vi "main.vi"() -> ()   [LabVIEW 2013]
panel:
  out "Array 2":string[](array[string])
  in  "Tab Control":enum32{"Page 1", "Page 2"}(tab)
  in  "Ring 2":u16(ring)
  in  "Ring":u16(ring)
  out "XY Graph":cluster{"X":dbl, "Y":dbl}[](graph)
  out "Waveform Chart":dbl(graph)
  in  "Listbox":i32(listbox)
  in  "Cluster":cluster{"String":string}
  in  "Array":dbl[](array[numeric])
  out "String 2":string
  in  "String":string
  out "Boolean 2":bool
  out "Numeric 2":dbl
  in  "Boolean":bool
  in  "Numeric":dbl
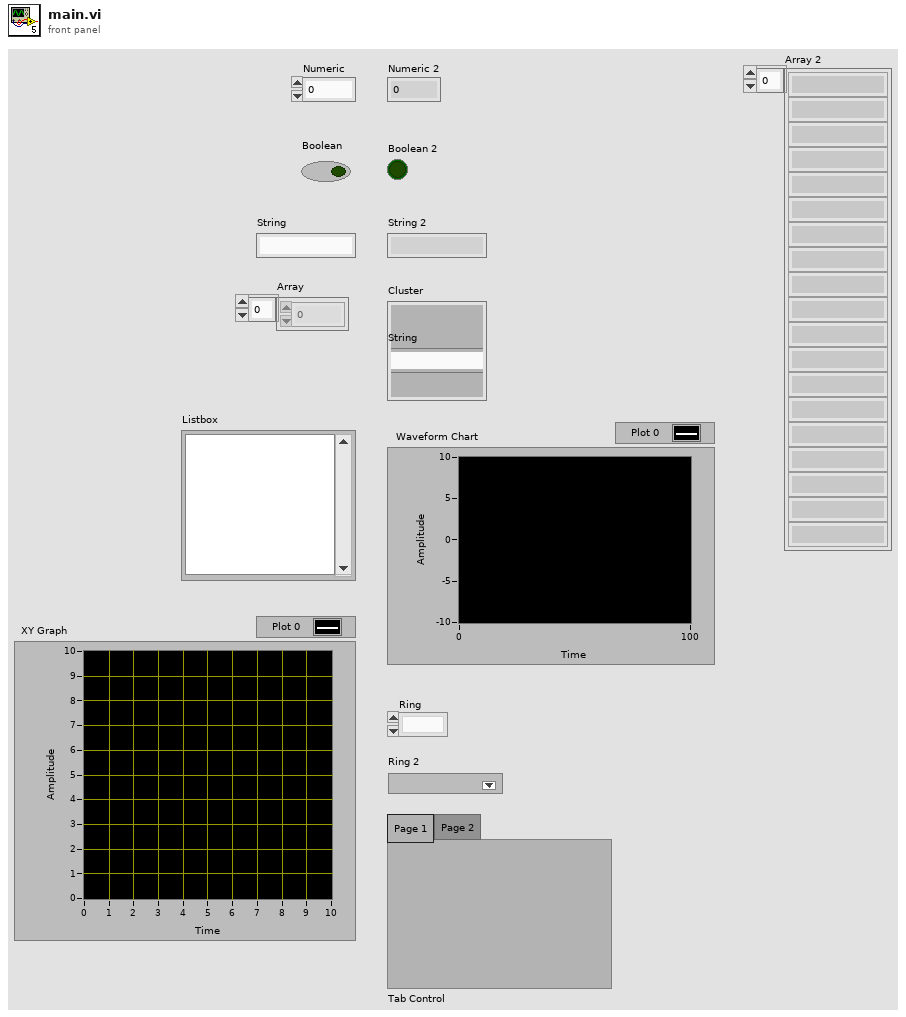
[diagram p1: front panel]
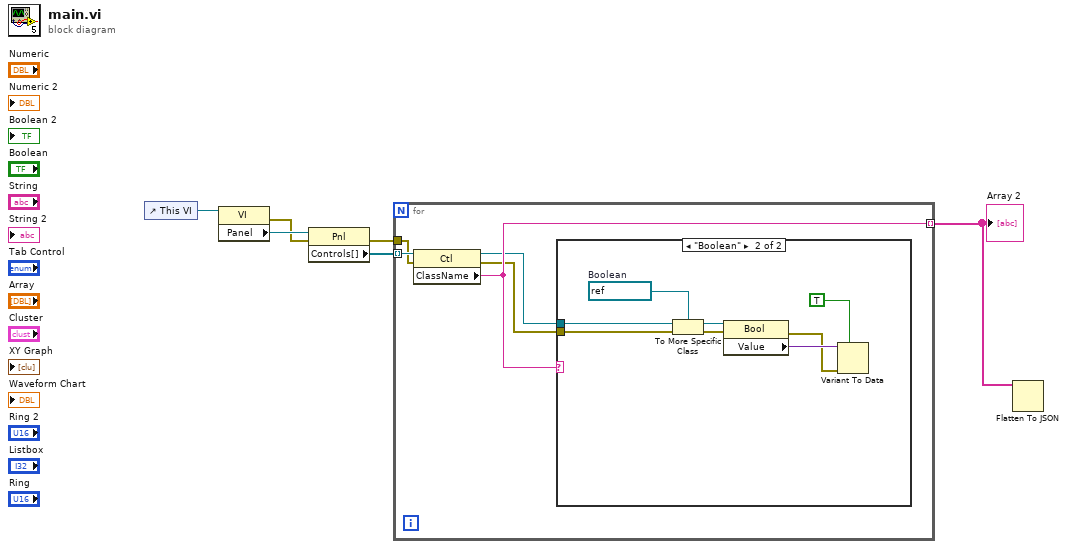
[diagram p0: block diagram]
diagram:
  n1 = control-ref of="This VI"() -> (w6:refnum<vi>)
  n2 = property class="VI"(reference=w6) -> (error out=w4:errorcluster, "Panel"=w5:refnum<vi>)  [unwired: 1 in, 1 out]
  n3 = property class="Pnl"(reference=w5, error in=w4) -> (error out=w2:errorcluster, "Controls[]"=w3:refnum<vi>[])  [unwired: 1 out]
  n4 = for {
    tunnel: w3 -> [w11] mode=indexing
    tunnel: w2 -> [w10]
    tunnel: [w9] -> w1 mode=indexing
    n5 = property class="Ctl"(reference=w11, error in=w10) -> (reference out=w8:refnum<vi>, error out=w7:errorcluster, "ClassName"=w9:string)
    n6 = case shown="\"Boolean\"" w9 {
      tunnel: w8 -> [_ w19]
      tunnel: w7 -> [_ w17]
      frame "\u0000", Default {
      }
      frame "Boolean" {
        w18 = refnum<vi> refnum  # Boolean
        n7 = To More Specific Class(target class=w18, reference=w19, error in=w17) -> (specific class reference=w16:refnum<vi>, error out=w15:errorcluster)
        n8 = property class="Bool"(reference=w16, error in=w15) -> (error out=w12:errorcluster, "Value"=w14:variant)  [unwired: 1 out]
        n9 = Variant To Data(error in=w12, type=TRUE, Variant=w14) -> ()  [unwired: 2 out]
      }
    }
  }
  "Array 2" <- w1
  n10 = Flatten To JSON(anything=w1) -> ()  [unwired: 2 in, 2 out]
